vi "Dynamic Events.vi"() -> ()   [LabVIEW 2021]
panel:
  in  "String":string
  # "Dynamic Events"
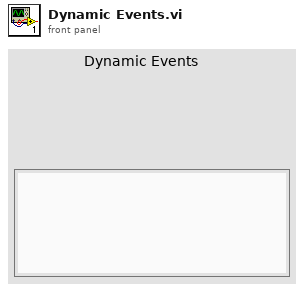
[diagram p1: front panel]
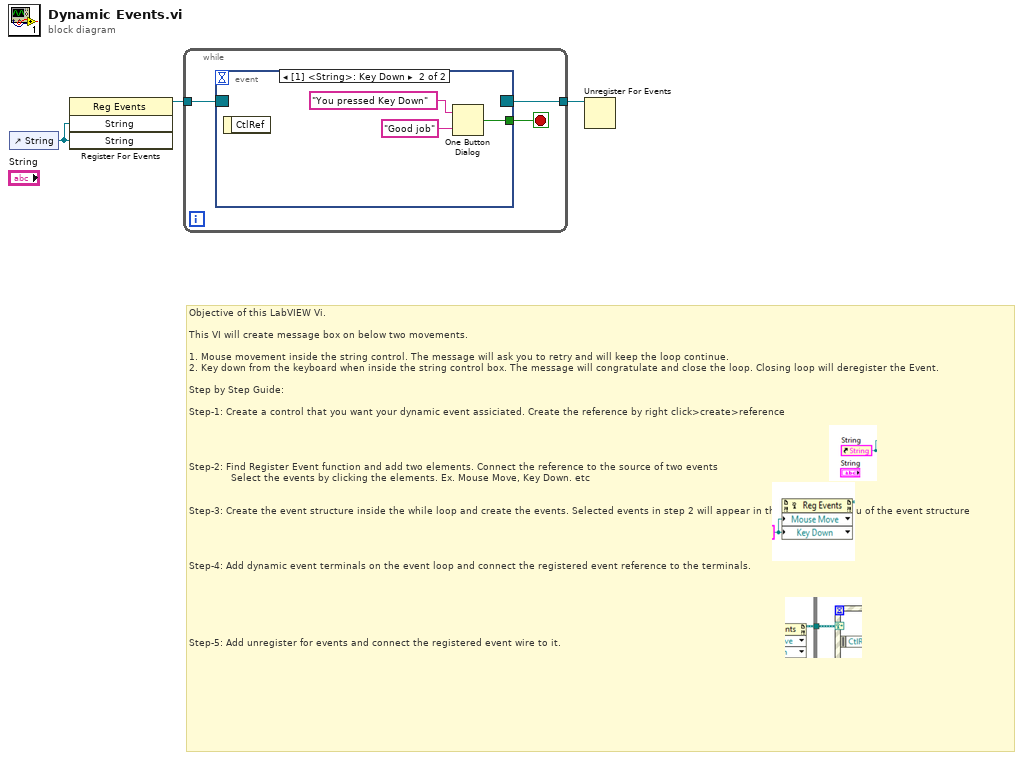
[diagram p0: block diagram]
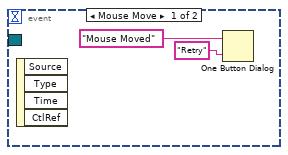
[diagram p2: hidden frame]
diagram:
  # "Objective of this LabVIEW Vi. \n\nThis VI will create message box on below two movements.\n\n1. Mouse movement inside the string control. The message will ask you to retry and will keep the loop continue. \n2. Key down from the keyboard when inside the string control box. The message will congratulate and close the loop. Closing loop will deregister the Event. \n\nStep by Step Guide:\n\nStep-1: Create a control that you want your dynamic event assiciated. Create the reference by right click>create>reference \n\n\n\n\nStep-2: Find Register Event function and add two elements. Connect the reference to the source of two events\n              Select the events by clicking the elements. Ex. Mouse Move, Key Down. etc\n\n\nStep-3: Create the event structure inside the while loop and create the events. Selected events in step 2 will appear in the add event menu of the event structure\n\n\n\n\nStep-4: Add dynamic event terminals on the event loop and connect the registered event reference to the terminals. \n\n\n\n\n\n\nStep-5: Add unregister for events and connect the registered event wire to it."
  n1 = control-ref of="String"() -> (w3:refnum<vi>)
  n2 = register-events(w3, w3) -> (reference out=w2:refnum<event-registration>)  [unwired: 2 in, 1 out]
  n3 = while {
    tunnel: w2 -> [w6]
    tunnel: [w5] -> w1
    stop <- w4 stop-if-true
    n4 = event shown="[1] <String>: Key Down" {
      selector: w6 -> [_ _]
      dyn-events: [_ _] -> w5
      timeout: _ -> [_ _]
      tunnel: [_ w9] -> w4
      event Mouse Move {
        n5 = event-data() -> ()  [unwired: 1 in, 4 out]
        n6 = One Button Dialog(message="Mouse Moved", button name ("OK")="Retry") -> ()  [unwired: 1 out]
      }
      event Key Down {
        n7 = event-data() -> ()  [unwired: 1 in, 1 out]
        n8 = One Button Dialog(message="You pressed Key Down", button name ("OK")="Good job") -> (true=w9:bool)
      }
    }
  }
  n9 = Unregister For Events(event registration refnum=w1) -> ()  [unwired: 1 in, 1 out]
